vi "Evaluate Polynomial with Matrix (DBL).vi"(2 "P(x)":dbl[](array[numeric]) min=0.0 max=127.0 format="%#.6g", 3 "A":T1) -> (0 "error":i32, 1 "P([A])":T1)   [LabVIEW 2017, in "NI_AALPro.lvlib"]
doc: "Evaluates the polynomial <B>P(x)</B> with matrix <B>A</B>. The data types you wire to the <B>P(x)</B> and <B>A</B> inputs determine the polymorphic instance to use."
uses:
  NI_AALPro.lvlib
  RealMatrix.ctl
  Real A x B.vi
  Add - RM,RM.vi
  Multiply - RM,R.vi
  Create Special Real Matrix.vi
  NI_AALBase.lvlib
  NI_Matrix.lvlib
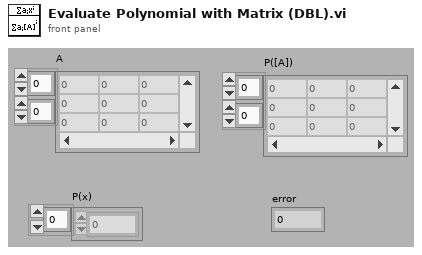
[diagram p1: front panel]
types:
  T1 = typedef "NI_Matrix.lvlib/RealMatrix.ctl" = dbl[][]
  T2 = enum32{"Identity", "Diagonal", "Toepliz", "Vandermonde", "Companion"}
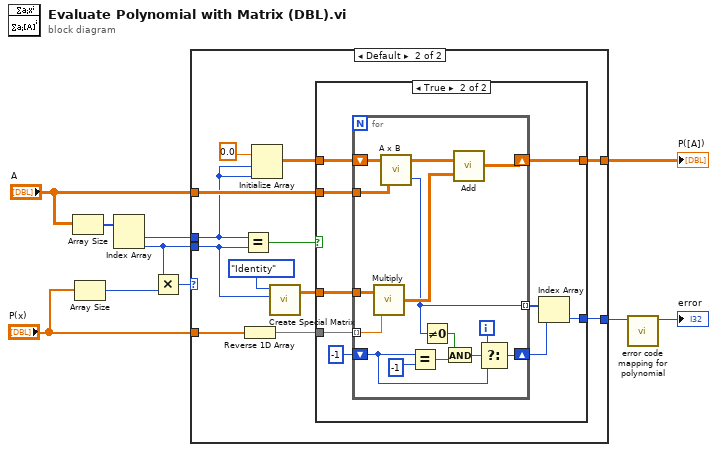
[diagram p0: block diagram]
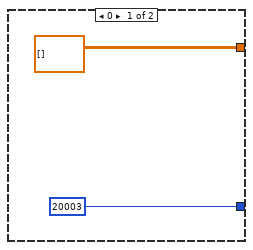
[diagram p2: hidden frame]
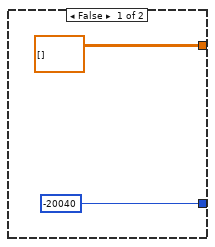
[diagram p3: hidden frame]
diagram:
  n1 = Array Size(array="A") -> (size(s)=w5:i32[])
  n2 = Array Size(array="P(x)") -> (size(s)=w7:i32)
  n3 = Index Array(array=w5) -> (element #1=w4:i32, element #2=w3:i32)  [unwired: 2 in]
  n4 = Multiply(x=w3, y=w7) -> (x*y=w6:i32)
  n5 = case shown="Default" w6 {
    tunnel: "A" -> [_ w18]
    tunnel: "P(x)" -> [_ w17]
    tunnel: [T1 [] ("A") w16] -> w9
    tunnel: [20003 ("empty array") w15] -> w2
    tunnel: w4 -> [_ w14]
    tunnel: w3 -> [_ w13]
    frame 0 {
    }
    frame Default {
      n6 = Equal?(x=w14, y=w13) -> (x = y?=w23:bool)
      n7 = Reverse 1D Array(array=w17) -> (reversed array=w24:dbl[])
      n8 = Initialize Array(0.0, w14, w14) -> (w21:dbl[][])
      n9 = call-poly "Create Special Matrix.vi"("matrix type"=T2."Identity", "matrix size"=w13) -> ("Special Matrix"=w20:T1)  [unwired: 3 in, 1 out]
      n10 = case shown="True" w23 {
        tunnel: w24 -> [_ w35]
        tunnel: w21 -> [_ w34]
        tunnel: w18 -> [_ w33]
        tunnel: w20 -> [_ w32]
        tunnel: [T1 [] ("A") w31] -> w16
        tunnel: [-20040 ("not a square matrix") w27] -> w15
        frame False {
        }
        frame True {
          n11 = for {
            shift-right: [w44] -> w31
            shift-left: w34 -> [w50]
            tunnel: w35 -> [w47] mode=indexing
            tunnel: w33 -> [w49]
            tunnel: w32 -> [w48]
            shift-right: [w39] -> w28
            shift-left: -1 -> [w37]
            tunnel: [w36] -> w29 mode=indexing
            i -> [w38]
            n12 = call-poly "Multiply.vi"("Real Scalar c"=w47, "Real Matrix A"=w48) -> ("A * c"=w46:T1)
            n13 = call-poly "A x B.vi"("B"=w49, "A"=w50) -> ("error"=w36:i32, "A x B"=w45:T1)
            n14 = Equal?(x=w37, y=-1) -> (x = y?=w41:bool)
            n15 = Not Equal To 0?(x=w36) -> (x != 0?=w42:bool)
            n16 = And(x=w42, y=w41) -> (x .and. y?=w40:bool)
            n17 = call-poly "Add.vi"("Real Matrix B"=w46, "Real Matrix A"=w45) -> ("A + B"=w44:T1)
            n18 = Select(t=w38, s=w40, f=w37) -> (s? t:f=w39:i32)
          }
          n19 = Index Array(array=w29, index=w28) -> (element=w27:i32)
        }
      }
    }
  }
  "P([A])" <- w9
  n20 = call "error code mapping for polynomial.vi"("error in"=w2) -> ("error out"=→"error":i32)  [unwired: 10 in]
